vi "FindUSBIResource.vi"(0 "error in (no error)":errorcluster) -> (1 "Ophir Resource":string, 2 "Ophir Board":string, 3 "Debug Index":i32, 4 "error out":errorcluster)   [LabVIEW 2012]
uses:
  <vilib>/Instr/_visa.llb/VISA Find Search Mode.ctl
panel:
  out "Debug STR":string
  out "Resource List":string[](array[string])
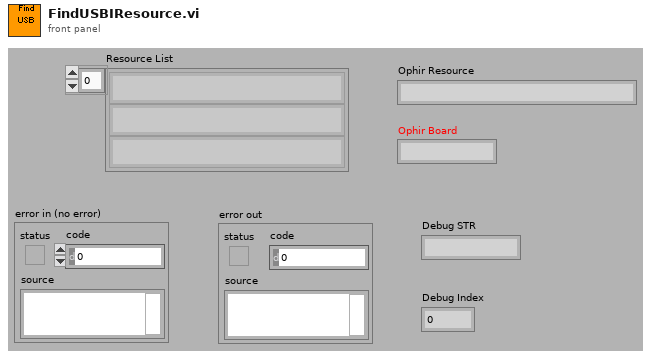
[diagram p1: front panel]
types:
  T1 = typedef "VISA Find Search Mode.ctl" = u32
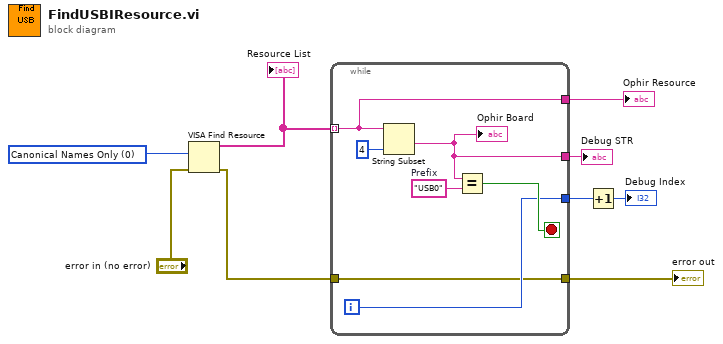
[diagram p0: block diagram]
diagram:
  w6 = T1 0 items=["Canonical Names Only"=0, "Aliases Only"=1, "Include Matching Aliases"=2, "Include All Aliases"=4] ("Search Mode")
  n1 = VISA Find Resource(8:"error in (no error)", 10:w6) -> (0:w2:errorcluster, 3:w9:string[])  [unwired: 1 in, 1 out]
  "Resource List" <- w9
  n2 = while {
    tunnel: w9 -> [w13] mode=indexing
    tunnel: [w10] -> w8
    tunnel: [w13] -> w4
    tunnel: [w12] -> w5
    tunnel: [w11] -> w3
    tunnel: w2 -> [w11]
    i -> [w12]
    stop <- w14 stop-if-true
    w15 = "USB0"  # Prefix
    n3 = String Subset(string=w13, length (rest)=4 ("length (rest)")) -> (substring=w10:string)  [unwired: 1 in]
    "Ophir Board" <- w10
    n4 = Equal?(x=w10, y=w15) -> (x = y?=w14:bool)
  }
  "Debug STR" <- w8
  "Ophir Resource" <- w4
  "error out" <- w3
  n5 = Increment(x=w5) -> (x+1=→"Debug Index":i32)
